vi "Main.vi"(11 "Module Admin":refnum<class "Delacor_lib_QMH_Cloneable Module Admin.lvclass">) -> ()   [LabVIEW 2020, in "Lock-in amplifier.lvlib"]
doc: "This template is based off of the Queued Message Handler design pattern and the Queued Message Handler project template that ships with LabVIEW.\n\nThe main difference is that the queue is private to this module and communication between modules is performed via Broadcast and Request events.\n\nRequest events are wrapped in public API methods and are handled in the Event Handling Loop (EHL) of this VI. Any module can register for Broadcast events sent by this module. The EHL generates messages based on user interface actions.\n\nThe Message Handling Loop (MHL) processes messages generated by the EHL, or by other messages. The messages are string values, so new messages can be added easily to the Message Cases case structure in the MHL. Each message cluster can also provide an optional value for Message Data, which is a variant that can be converted to whatever message-specific data is required.\n_____\nBased on DQMH Project Template 6.1.0.94.\n____\nPantherLAB Templates 1.0.0.1\nCopyright (c) 2022, PantherLAB\n____\nPantherLAB Templates 1.0.0.5\nCopyright (c) 2022, PantherLAB"
uses:
  Lock-in amplifier.lvlib
  <vilib>/Delacor/Delacor QMH/Libraries/Cloneable Module Admin_class/Delacor_lib_QMH_Cloneable Module Admin.lvclass
  C:/Program Files (x86)/National Instruments/LabVIEW 2020/vi.lib/Delacor/Delacor QMH/Libraries/Module Admin_class/Delacor_lib_QMH_Module Admin.lvclass
  Module Data--cluster.ctl
  Helper Loop Status--enum.ctl
  <vilib>/Delacor/Delacor QMH/Libraries/Cloneable Module Admin_class/Delacor_lib_QMH_Cloneable Module Admin.lvclass/Delacor_lib_QMH_Cloneable Module Admin.ctl
  <vilib>/Delacor/Delacor QMH/Libraries/Message Queue_class/Delacor_lib_QMH_Message Queue.lvclass/Delacor_lib_QMH_Message Queue.ctl
  Stop Argument--cluster.ctl
  <vilib>/Delacor/Delacor QMH/Libraries/Module Admin_class/Delacor_lib_QMH_Module Admin.lvclass/Delacor_lib_QMH_Module Admin.ctl
  Draw Panel into Subpanel Argument--cluster.ctl
  Remove Panel from Subpanel Argument--cluster.ctl
  <vilib>/Utility/miscctls.llb/LVPointTypeDef.ctl
  <vilib>/Delacor/Delacor QMH/Libraries/Cloneable Module Admin_class/Delacor_lib_QMH_Get Module ID.vi
  <vilib>/Delacor/Delacor QMH/Libraries/Message Queue_class/Delacor_lib_QMH_Enqueue Message (Single).vi
  <vilib>/Delacor/Delacor QMH/Libraries/Module Admin_class/Delacor_lib_QMH_Get External Launch.vi
  <vilib>/Utility/error.llb/Error Cluster From Error Code.vi
  <vilib>/ErrorRing/Error Ring.xnode
  <vilib>/Delacor/Delacor QMH/Libraries/Message Queue_class/Delacor_lib_QMH_Message Queue.lvclass
  Local Events/Local Events.lvlib
panel:
  out "error out":errorcluster
  out "Status":string
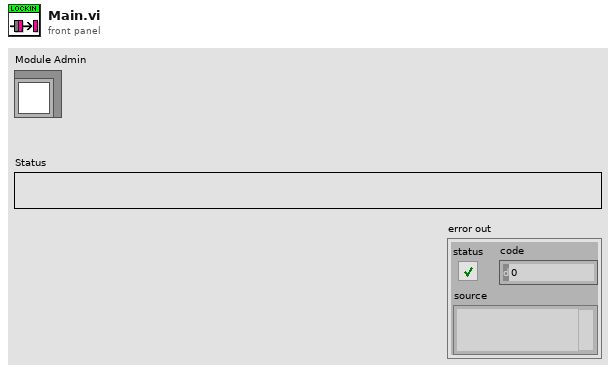
[diagram p1: front panel]
types:
  T1 = typedef "Lock-in amplifier.lvlib/Request Events--cluster.ctl" = cluster{"Stop Module":refnum<user-event>, "Show Panel":refnum<user-event>, "Hide Panel":refnum<user-event>, "Show Diagram":refnum<user-event>, "Get Module Execution Status":refnum<user-event>, "Draw Panel into Subpanel":refnum<user-event>, "Remove Panel from Subpanel":refnum<user-event>}
  T2 = typedef "Lock-in amplifier.lvlib/Local Events.lvlib/Local Events--cluster.ctl" = cluster{"Wake up Helper Loop":refnum<user-event>, "Put Helper Loop to Sleep":refnum<user-event>}
  T3 = typedef "Lock-in amplifier.lvlib/Module Data--cluster.ctl" = cluster{"Status":string, "SubPanel":refnum<vi>, "Panel Status":bool}
  T4 = typedef "Lock-in amplifier.lvlib/Helper Loop Status--enum.ctl" = enum16{"Awake", "Asleep"}
  T5 = enum32{"invalid lock state", "Not Locked", "Locked (No Password)", "Password-protected"}
  T6 = typedef "Lock-in amplifier.lvlib/Stop Argument--cluster.ctl" = cluster{"Module ID":i32, "Origin":string, "Exit via Stop Module Req?":bool, "Wait for Module to stop?":bool}
  T7 = typedef "Lock-in amplifier.lvlib/Draw Panel into Subpanel Argument--cluster.ctl" = cluster{"Module ID":i32, "Sub Panel":refnum<vi>}
  T8 = typedef "Lock-in amplifier.lvlib/Remove Panel from Subpanel Argument--cluster.ctl" = cluster{"Module ID":i32, "Boolean":bool}
  T9 = typedef "LVPointTypeDef.ctl" = cluster{"Horizontal":i16, "Vertical":i16}
  T10 = enum32{"Invalid", "Standard", "Closed", "Hidden", "Minimized", "Maximized"}
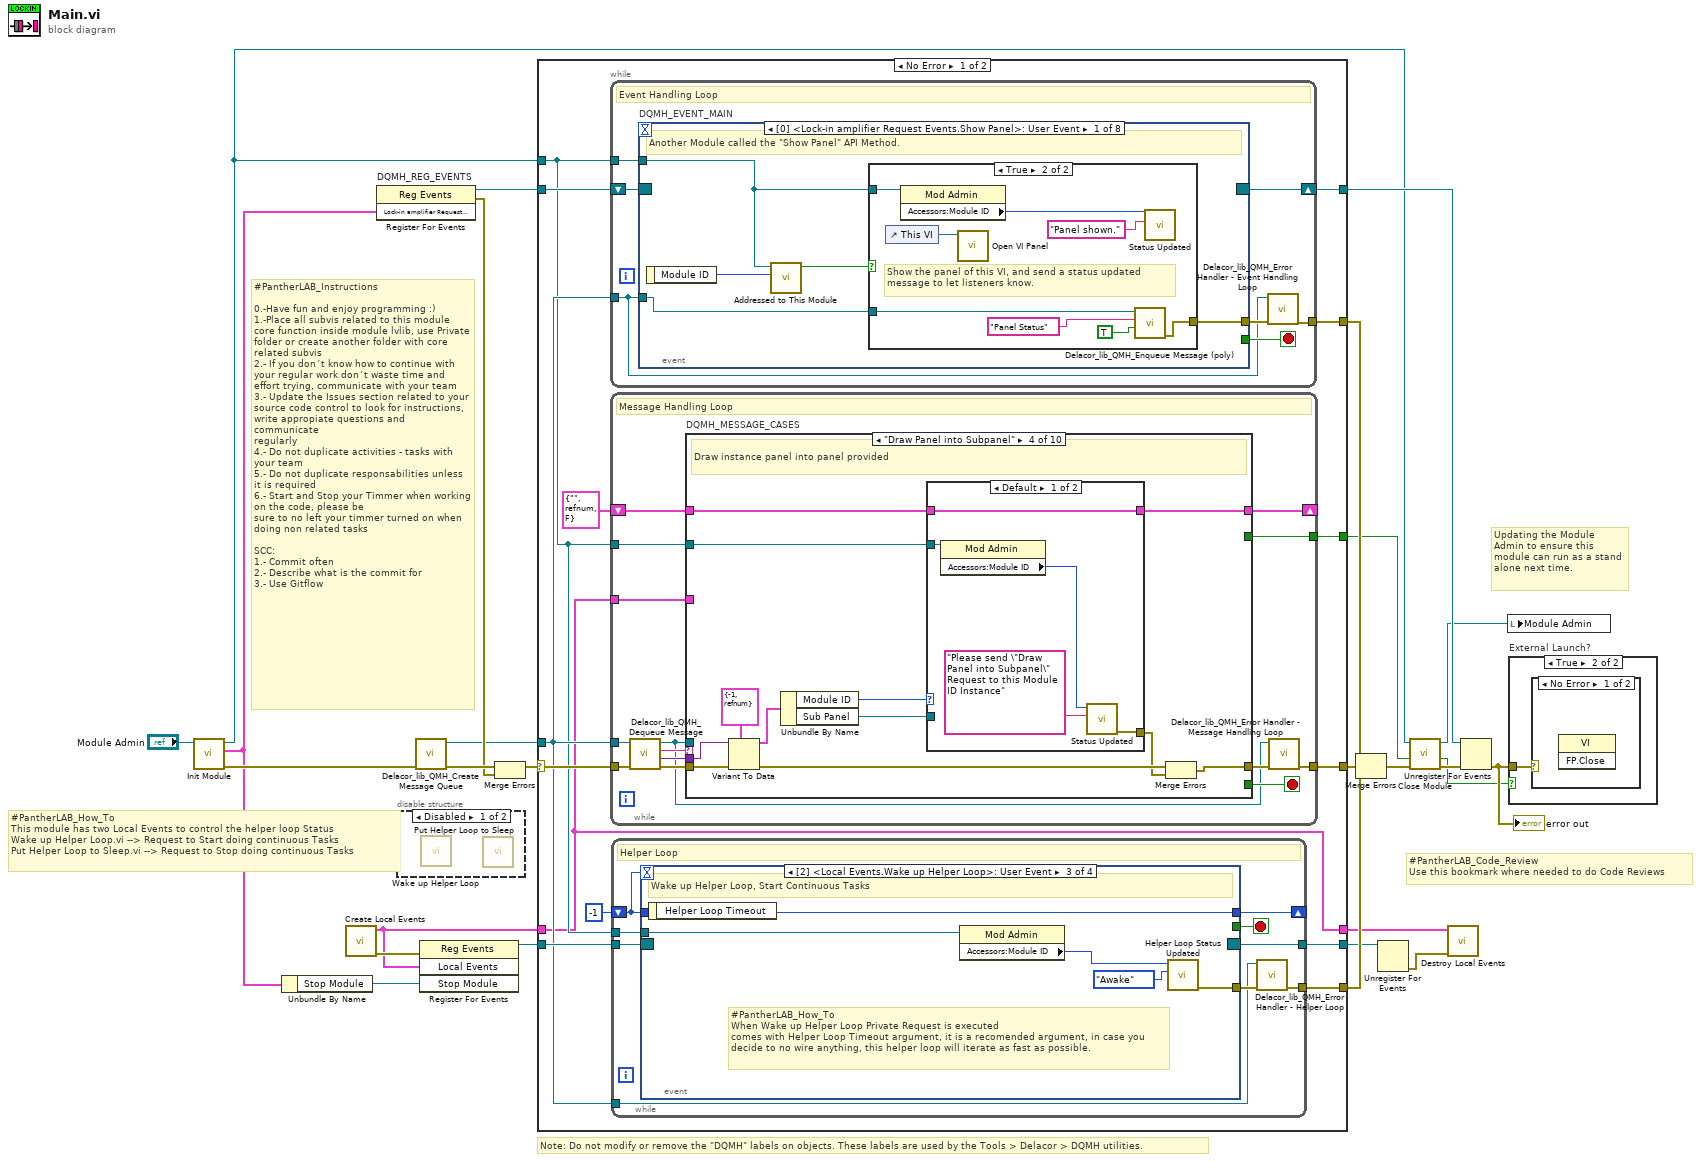
[diagram p0: block diagram]
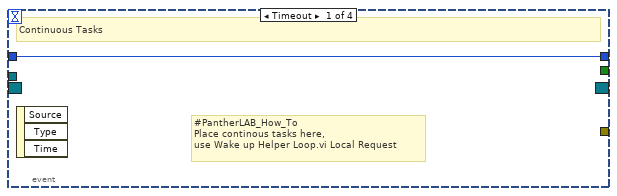
[diagram p3: hidden frame]
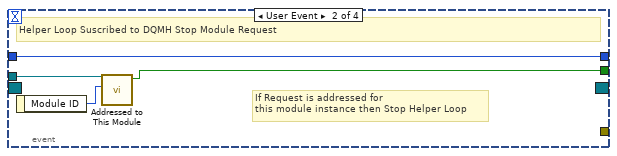
[diagram p4: hidden frame]
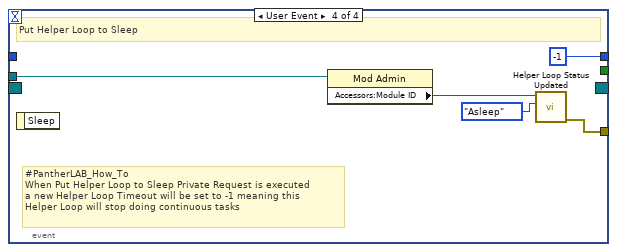
[diagram p5: hidden frame]
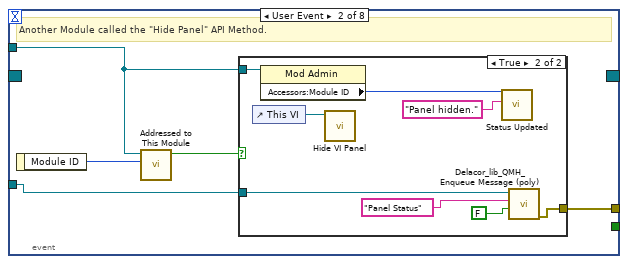
[diagram p7: hidden frame]
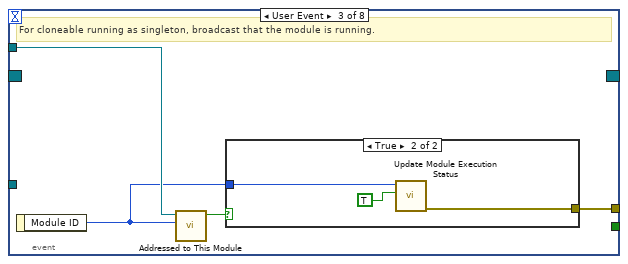
[diagram p9: hidden frame]
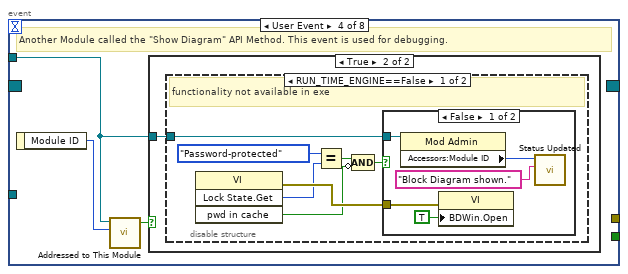
[diagram p11: hidden frame]
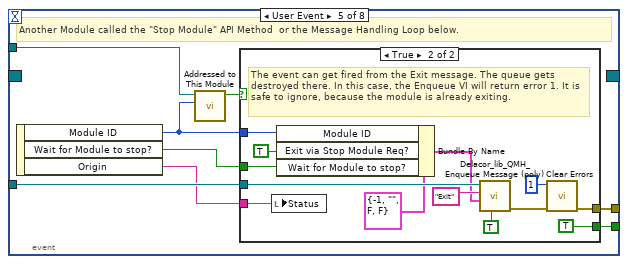
[diagram p15: hidden frame]
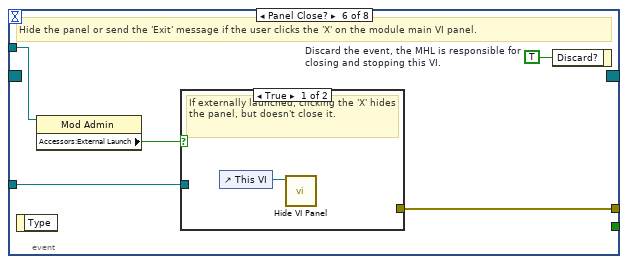
[diagram p17: hidden frame]
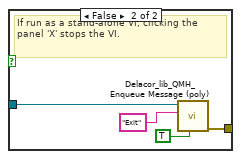
[diagram p18: hidden frame]
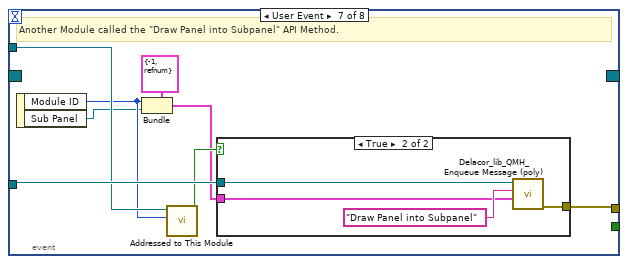
[diagram p19: hidden frame]
diagram:
  # "#PantherLAB_How_To\nThis module has two Local Events to control the helper loop Status\nWake up Helper Loop.vi --> Request to Start doing continuous Tasks\nPut Helper Loop to Sleep.vi --> Request to Stop doing continuous Tasks"
  # "#PantherLAB_Code_Review\nUse this bookmark where needed to do Code Reviews"
  # "#PantherLAB_Instructions\n\n0.-Have fun and enjoy programming :)\n1.-Place all subvis related to this module core function inside module lvlib, use Private folder or create another folder with core related subvis \n2.- If you don´t know how to continue with your regular work don´t waste time and effort trying, communicate with your team\n3.- Update the Issues section related to your source code control to look for instructions, write appropiate questions and communicate\nregularly\n4.- Do not duplicate activities - tasks with your team\n5.- Do not duplicate responsabilities unless it is required\n6.- Start and Stop your Timmer when working on the code, please be\nsure to no left your timmer turned on when doing non related tasks\n\nSCC:\n1.- Commit often\n2.- Describe what is the commit for\n3.- Use Gitflow"
  # "Note: Do not modify or remove the \"DQMH\" labels on objects. These labels are used by the Tools > Delacor > DQMH utilities."
  # "Updating the Module Admin to ensure this module can run as a stand alone next time."
  n1 = call "Init Module.vi"("Cloneable Module Admin in"="Module Admin") -> ("error out"=w23:errorcluster, "Lock-in amplifier Request Events"=w4:T1, "Cloneable Module Admin out"=w10:refnum<class "Delacor_lib_QMH_Cloneable Module Admin.lvclass">)  [unwired: 8 in]
  n2 = Unbundle By Name(w4) -> ("Stop Module"=w3:refnum<user-event>)
  n3 = call "Create Local Events.vi"() -> ("error out"=w16:errorcluster, "Local Events"=w2:T2)  [unwired: 10 in]
  n4 = register-events "DQMH_REG_EVENTS"(w4) -> (reference out=w13:refnum<event-registration>, error out=w18:errorcluster)  [unwired: 2 in]
  n5 = disable-structure shown="Disabled" {
    frame Disabled {
      n6 = call "Wake up Helper Loop.vi"() -> ()  [unwired: 11 in, 1 out]
      n7 = call "Put Helper Loop to Sleep.vi"() -> ()  [unwired: 11 in, 1 out]
    }
    frame Enabled {
    }
  }
  n8 = call <vilib>:"Delacor_lib_QMH_Create Message Queue.vi"("error in"=w23) -> ("error out"=w20:errorcluster, "Message Queue"=w12:refnum<class "Delacor_lib_QMH_Message Queue.lvclass">)  [unwired: 9 in]
  n9 = register-events(error in=w16, w2, w3) -> (reference out=w5:refnum<event-registration>)  [unwired: 1 in, 1 out]
  n10 = Merge Errors(w20, w18) -> (w19:errorcluster)
  n11 = case shown="No Error" w19 {
    selector: w19 -> [w38 w326]
    tunnel: [w40 w325] -> w24
    tunnel: [w36 w324] -> w14
    tunnel: w13 -> [w34 w324]
    tunnel: w12 -> [w29 w317]
    tunnel: [w39 _] -> w25
    tunnel: w10 -> [w28 w320]
    tunnel: [w33 _] -> w8
    tunnel: [w32 w316] -> w6
    tunnel: w5 -> [w31 w316]
    tunnel: [w37 _] -> w17
    tunnel: w2 -> [w27 w315]
    tunnel: [w27 w315] -> w1
    frame No Error {
      n12 = while {
        tunnel: w29 -> [w65]
        shift-right: [w68] -> w36
        shift-left: w34 -> [w69]
        tunnel: [w70] -> w39
        tunnel: w28 -> [w66]
        stop <- w67 stop-if-true
        # "Event Handling Loop"
        n13 = event "DQMH_EVENT_MAIN" shown="[0] <Lock-in amplifier Request Events.Show Panel>: User Event" {
          selector: w69 -> [_ _ _ _ _ _ _ _]
          dyn-events: [_ _ _ _ _ _ _ _] -> w68
          timeout: _ -> [_ _ _ _ _ _ _ _]
          tunnel: [_ _ _ _ w124 _ _ _] -> w67
          tunnel: w65 -> [w72 w85 _ _ w127 w143 w158 w170]
          tunnel: [w76 w89 w101 _ w128 w146 w159 w171] -> w71
          tunnel: w66 -> [w73 w86 w99 w105 w126 w144 w156 w168]
          event User Event {
            # "Another Module called the \"Show Panel\" API Method."
            n14 = event-data() -> ("Module ID"=w74:i32)  [unwired: 1 in]
            n15 = call "Addressed to This Module.vi"("Module ID from Argument"=w74, "Module Admin"=w73) -> ("Addressed to this instance?"=w75:bool)  [unwired: 8 in, 1 out]
            n16 = case shown="True" w75 {
              tunnel: w73 -> [_ w81]
              tunnel: w72 -> [_ w79]
              tunnel: [_ w84] -> w76
              frame False {
              }
              frame True {
                # "Show the panel of this VI, and send a status updated message to let listeners know."
                n17 = control-ref of="This VI"() -> (w83:refnum<vi>)
                n18 = property class="Mod Admin"(reference=w81) -> ("Accessors:Module ID"=w80:i32)  [unwired: 1 in, 2 out]
                n19 = call "Open VI Panel.vi"("VI"=w83) -> ()  [unwired: 10 in, 1 out]
                n20 = call-poly <vilib>:"Delacor_lib_QMH_Enqueue Message (poly).vi"("Message Data"=TRUE, "Message"="Panel Status" ("format string"), "Message Queue in"=w79) -> ("error out"=w84:errorcluster)  [unwired: 7 in, 1 out]
                n21 = call "Status Updated.vi"("Status"="Panel shown." ("format string"), "Module ID"=w80) -> ()  [unwired: 9 in, 1 out]
              }
            }
          }
          event User Event {
            # "Another Module called the \"Hide Panel\" API Method."
            n22 = event-data() -> ("Module ID"=w87:i32)  [unwired: 1 in]
            n23 = call "Addressed to This Module.vi"("Module ID from Argument"=w87, "Module Admin"=w86) -> ("Addressed to this instance?"=w88:bool)  [unwired: 8 in, 1 out]
            n24 = case shown="True" w88 {
              tunnel: w86 -> [_ w94]
              tunnel: w85 -> [_ w90]
              tunnel: [_ w97] -> w89
              frame False {
              }
              frame True {
                n25 = control-ref of="This VI"() -> (w96:refnum<vi>)
                n26 = property class="Mod Admin"(reference=w94) -> ("Accessors:Module ID"=w93:i32)  [unwired: 1 in, 2 out]
                n27 = call "Hide VI Panel.vi"("VI"=w96) -> ()  [unwired: 10 in, 1 out]
                n28 = call "Status Updated.vi"("Status"="Panel hidden." ("format string"), "Module ID"=w93) -> ()  [unwired: 9 in, 1 out]
                n29 = call-poly <vilib>:"Delacor_lib_QMH_Enqueue Message (poly).vi"("Message Data"=FALSE, "Message"="Panel Status" ("format string"), "Message Queue in"=w90) -> ("error out"=w97:errorcluster)  [unwired: 7 in, 1 out]
              }
            }
          }
          event User Event {
            # "For cloneable running as singleton, broadcast that the module is running."
            n30 = event-data() -> ("Module ID"=w98:i32)  [unwired: 1 in]
            n31 = call "Addressed to This Module.vi"("Module ID from Argument"=w98, "Module Admin"=w99) -> ("Addressed to this instance?"=w100:bool)  [unwired: 8 in, 1 out]
            n32 = case shown="True" w100 {
              tunnel: [_ w104] -> w101
              tunnel: w98 -> [_ w103]
              frame False {
              }
              frame True {
                n33 = call "Update Module Execution Status.vi"("Running?"=TRUE, "Module ID"=w103) -> ("error out"=w104:errorcluster)  [unwired: 9 in]
              }
            }
          }
          event User Event {
            # "Another Module called the \"Show Diagram\" API Method. This event is used for debugging."
            n34 = event-data() -> ("Module ID"=w106:i32)  [unwired: 1 in]
            n35 = call "Addressed to This Module.vi"("Module ID from Argument"=w106, "Module Admin"=w105) -> ("Addressed to this instance?"=w107:bool)  [unwired: 8 in, 1 out]
            n36 = case shown="True" w107 {
              tunnel: w105 -> [_ w108]
              frame False {
              }
              frame True {
                n37 = disable-structure shown="RUN_TIME_ENGINE==False" {
                  disable-tunnel: w108 -> [w109 _]
                  frame condition #0 (active) {
                    # "functionality not available in exe"
                    n38 = invoke class="VI" method="Lock State.Get"() -> (error out=w115:errorcluster, "Get Lock State"=w114:T5, "pwd in cache"=w111:bool)  [unwired: 4 in, 1 out]
                    n39 = Equal?(x=T5."Password-protected", y=w114) -> (x = y?=w112:bool)
                    n40 = Compound Arithmetic op=AND(w112, invert w111) -> (w110:bool)
                    n41 = case shown="False" w110 {
                      tunnel: w115 -> [w120 _]
                      tunnel: w109 -> [w117 _]
                      frame False {
                        n42 = property class="Mod Admin"(reference=w117) -> ("Accessors:Module ID"=w116:i32)  [unwired: 1 in, 2 out]
                        n43 = property class="VI"(error in=w120, "BDWin.Open"=TRUE ("Block Diagram Window:Open")) -> ()  [unwired: 1 in, 2 out]
                        n44 = call "Status Updated.vi"("Status"="Block Diagram shown." ("format string"), "Module ID"=w116) -> ()  [unwired: 9 in, 1 out]
                      }
                      frame True {
                        # "Password-protected VI, and the password is not in the cache. Do not show the diagram."
                      }
                    }
                  }
                  frame condition #1 {
                  }
                }
              }
            }
          }
          event User Event {
            # "Another Module called the \"Stop Module\" API Method  or the Message Handling Loop below."
            n45 = event-data() -> ("Module ID"=w122:i32, "Wait for Module to stop?"=w123:bool, "Origin"=w121:string)  [unwired: 1 in]
            n46 = call "Addressed to This Module.vi"("Module ID from Argument"=w122, "Module Admin"=w126) -> ("Addressed to this instance?"=w125:bool)  [unwired: 8 in, 1 out]
            n47 = case shown="True" w125 {
              tunnel: [_ w140] -> w128
              tunnel: w127 -> [_ w136]
              tunnel: [_ TRUE] -> w124
              tunnel: w123 -> [_ w131]
              tunnel: w122 -> [_ w133]
              tunnel: w121 -> [_ w129]
              frame False {
              }
              frame True {
                # "The event can get fired from the Exit message. The queue gets destroyed there. In this case, the Enqueue VI will return error 1. It is safe to ignore, because the module is already exiting."
                n48 = local write "Status"(w129) -> ()
                n49 = Bundle By Name(cluster=T6 {"Module ID"=-1, "Origin"="", "Exit via Stop Module Req?"=FALSE, "Wait for Module to stop?"=FALSE} ("Stop Argument"), "Module ID"=w133, "Exit via Stop Module Req?"=TRUE, "Wait for Module to stop?"=w131) -> (w130:T6)
                n50 = call-poly <vilib>:"Delacor_lib_QMH_Enqueue Message (poly).vi"("Priority Message? (F)"=TRUE, "Message Data"=w130, "Message"="Exit", "Message Queue in"=w136) -> ("error out"=w141:errorcluster)  [unwired: 6 in, 1 out]
                n51 = call <vilib>:"Clear Errors.vi"("error in (no error)"=w141, "specific error code to clear (0: all)"=1) -> ("error out"=w140:errorcluster)  [unwired: 4 in, 1 out]
              }
            }
          }
          event Panel Close? {
            w145 = TRUE  # Discard the event, the MHL is responsible for closing and stopping this VI.
            # "Hide the panel or send the 'Exit' message if the user clicks the 'X' on the module main VI panel."
            n52 = event-data() -> ()  [unwired: 1 in, 1 out]
            n53 = property class="Mod Admin"(reference=w144) -> ("Accessors:External Launch"=w142:bool)  [unwired: 1 in, 2 out]
            n54 = case shown="True" w142 {
              tunnel: w143 -> [_ w150]
              tunnel: [_ w151] -> w146
              frame True {
                # "If externally launched, clicking the 'X' hides the panel, but doesn't close it."
                n55 = control-ref of="This VI"() -> (w147:refnum<vi>)
                n56 = call "Hide VI Panel.vi"("VI"=w147) -> ()  [unwired: 10 in, 1 out]
              }
              frame False {
                # "If run as a stand-alone VI, clicking the panel 'X' stops the VI."
                n57 = call-poly <vilib>:"Delacor_lib_QMH_Enqueue Message (poly).vi"("Priority Message? (F)"=TRUE, "Message"="Exit", "Message Queue in"=w150) -> ("error out"=w151:errorcluster)  [unwired: 7 in, 1 out]
              }
            }
            n58 = event-data("Discard?"=w145) -> ()  [unwired: 1 in, 1 out]
          }
          event User Event {
            # "Another Module called the \"Draw Panel into Subpanel\" API Method."
            n59 = event-data() -> ("Module ID"=w153:i32, "Sub Panel"=w152:refnum<vi>)  [unwired: 1 in]
            n60 = Bundle(cluster=T7 {"Module ID"=-1, "Sub Panel"=refnum} ("Draw Panel into Subpanel Argument"), "Module ID"=w153, "Sub Panel"=w152) -> (w154:T7)
            n61 = call "Addressed to This Module.vi"("Module ID from Argument"=w153, "Module Admin"=w156) -> ("Addressed to this instance?"=w157:bool)  [unwired: 8 in, 1 out]
            n62 = case shown="True" w157 {
              tunnel: w158 -> [_ w162]
              tunnel: w154 -> [_ w160]
              tunnel: [_ w163] -> w159
              frame False {
              }
              frame True {
                n63 = call-poly <vilib>:"Delacor_lib_QMH_Enqueue Message (poly).vi"("Message Data"=w160, "Message"="Draw Panel into Subpanel", "Message Queue in"=w162) -> ("error out"=w163:errorcluster)  [unwired: 7 in, 1 out]
              }
            }
          }
          event User Event {
            # "Another Module called the \"Remove Panel from Subpanel\" API Method."
            n64 = event-data() -> ("Module ID"=w165:i32, "Boolean"=w164:bool)  [unwired: 1 in]
            n65 = Bundle(cluster=T8 {"Module ID"=-1, "Boolean"=FALSE} ("Remove Panel from Subpanel Argument"), "Module ID"=w165, "Boolean"=w164) -> (w166:T8)
            n66 = call "Addressed to This Module.vi"("Module ID from Argument"=w165, "Module Admin"=w168) -> ("Addressed to this instance?"=w169:bool)  [unwired: 8 in, 1 out]
            n67 = case shown="True" w169 {
              tunnel: w170 -> [_ w174]
              tunnel: w166 -> [_ w172]
              tunnel: [_ w175] -> w171
              frame False {
              }
              frame True {
                n68 = call-poly <vilib>:"Delacor_lib_QMH_Enqueue Message (poly).vi"("Message Data"=w172, "Message"="Remove Panel from Subpanel", "Message Queue in"=w174) -> ("error out"=w175:errorcluster)  [unwired: 7 in, 1 out]
              }
            }
          }
        }
        n69 = call-dynamic "Delacor_lib_QMH_Error Handler - Event Handling Loop.vi"("error in"=w71, "Message Queue in"=w65) -> ("dup error in"=w70:errorcluster)  [unwired: 8 in, 1 out]
      }
      n70 = while {
        tunnel: w29 -> [w180]
        shift-right: [w184] -> _
        shift-left: T3 {"Status"="", "SubPanel"=refnum, "Panel Status"=FALSE} ("Data Cluster") -> [w185]
        tunnel: w38 -> [w188]
        tunnel: [w186] -> w40
        tunnel: w28 -> [w178]
        tunnel: [w177] -> w33
        tunnel: w27 -> [w176]
        stop <- w183 stop-if-true
        # "Message Handling Loop"
        n71 = call-dynamic "Delacor_lib_QMH_Dequeue Message.vi"("error in"=w188, "Message Queue in"=w180) -> ("error out"=w187:errorcluster, "Message Data"=w181:variant, "Message"=w182:string, "Message Queue out"=w179:refnum<class "Delacor_lib_QMH_Message Queue.lvclass">)  [unwired: 6 in]
        n72 = case "DQMH_MESSAGE_CASES" shown="\"Draw Panel into Subpanel\"" w182 {
          selector: w182 -> [_ _ _ _ _ _ _ _ _ w302]
          tunnel: w179 -> [_ _ _ _ _ _ _ w266 w292 _]
          tunnel: w187 -> [w208 w212 w219 w231 w250 w262 w264 w275 w298 w304]
          tunnel: [w206 w212 w218 w229 w249 w261 w264 w271 w295 w305] -> w189
          tunnel: w185 -> [w199 w211 w217 w222 w244 w260 w263 w270 w283 w303]
          tunnel: [w198 w211 w214 w221 w244 w260 w263 w270 w283 w303] -> w184
          tunnel: [_ _ _ _ _ _ _ _ w291 _] -> w183
          tunnel: w181 -> [_ _ w216 w227 w248 _ _ w269 w289 _]
          tunnel: w178 -> [w193 _ _ w220 w243 _ _ w268 w285 w300]
          tunnel: [_ _ _ _ _ _ _ _ w287 _] -> w177
          tunnel: w176 -> [_ _ _ _ _ _ _ _ _ _]
          frame "Initialize" {
            w190 = "Initial Message" ("Initial Message")
            # "#CodeNeeded - Initialize the appearance of the front panel."
            # "#CodeNeeded - Initialize your state data here."
            # "Initialize - Any operation that needs to be done before the module can receive messages. Synchronize Caller Events.vi will inform Start Module.vi that the module has launched and is ready to receive messages. Module Did Init.vi will broadcast that the module initialized."
            n73 = call "Synchronize Caller Events.vi"("error in (no error)"=w208, "Module Admin"=w193) -> ("error out"=w207:errorcluster, "Module Admin out"=w192:refnum<class "Delacor_lib_QMH_Cloneable Module Admin.lvclass">)  [unwired: 8 in]
            n74 = property class="Mod Admin"(reference=w192) -> ("Accessors:Module ID"=w195:i32, "Accessors:External Launch"=w194:bool)  [unwired: 1 in, 2 out]
            n75 = call "Module Name--constant.vi"("Module ID"=w195) -> ("Module Name"=w203:string)  [unwired: 10 in]
            n76 = property class="VI"("Front Panel.Title"=w203) -> (reference out=w205:refnum<vi>, error out=w210:errorcluster)  [unwired: 2 in]
            n77 = Select(t=T10."Hidden" ("State"), s=w194, f=T10."Standard" ("State")) -> (s? t:f=w200:T10)
            n78 = invoke class="VI" method="FP.Open"(reference=w205, error in=w210, "State"=w200) -> (reference out=w204:refnum<vi>, error out=w209:errorcluster)  [unwired: 2 in, 3 out]
            n79 = call "Module Name--constant.vi"("Module ID"=w195) -> ("Module Name"=w196:string)  [unwired: 10 in]
            n80 = Bundle By Name(cluster=w199, "Status"=w190) -> (w198:T3)
            n81 = invoke class="VI" method="FP.Center"(reference=w204, error in=w209) -> ()  [unwired: 1 in, 3 out]
            n82 = property on="Pane" class="Pane"("Origin"=T9 {"Horizontal"=0, "Vertical"=0}) -> ()  [unwired: 2 in, 2 out]
            n83 = call "Module Did Init.vi"("error in (no error)"=w207, "Initialized?"=TRUE, "Origin"=w196, "Module ID"=w195) -> ("error out"=w206:errorcluster)  [unwired: 7 in]
            "Status" <- w190
          }
          frame "---Module Specific---" {
            # "Separator -- The following cases handle messages specific to this Module."
          }
          frame "Panel Status" {
            n84 = Variant To Data(error in=w219, type=TRUE, Variant=w216) -> (data=w213:bool, error out=w218:errorcluster)
            n85 = Bundle By Name(cluster=w217, "Panel Status"=w213) -> (w214:T3)
          }
          frame "Draw Panel into Subpanel" {
            # "Draw instance panel into panel provided"
            n86 = Variant To Data(error in=w231, type=T7 {"Module ID"=-1, "Sub Panel"=refnum} ("Draw Panel into Subpanel Argument"), Variant=w227) -> (data=w225:T7, error out=w230:errorcluster)
            n87 = Unbundle By Name(w225) -> ("Module ID"=w223:i32, "Sub Panel"=w224:refnum<vi>)
            n88 = case shown="Default" w223 {
              tunnel: w224 -> [_ w241]
              tunnel: [w236 w242] -> w228
              tunnel: w222 -> [w234 w239]
              tunnel: [w234 w238] -> w221
              tunnel: w220 -> [w233 _]
              frame Default {
                n89 = property class="Mod Admin"(reference=w233) -> ("Accessors:Module ID"=w232:i32)  [unwired: 1 in, 2 out]
                n90 = call "Status Updated.vi"("Status"="Please send \"Draw Panel into Subpanel\" Request to this Module ID Instance", "Module ID"=w232) -> ("error out"=w236:errorcluster)  [unwired: 9 in]
              }
              frame 0.. {
                n91 = control-ref of="This VI"() -> (w240:refnum<vi>)
                n92 = call "Draw Panel into Subpanel Procedure.vi"("SubPanel in"=w241, "This VI"=w240) -> ("error out"=w242:errorcluster, "SubPanel out"=w237:refnum<vi>)  [unwired: 8 in]
                n93 = Bundle By Name(cluster=w239, "SubPanel"=w237) -> (w238:T3)
              }
            }
            n94 = Merge Errors(w230, w228) -> (w229:errorcluster)
          }
          frame "Remove Panel from Subpanel" {
            # "Remove panel from subpanel"
            n95 = Variant To Data(error in=w250, type=T8 {"Module ID"=-1, "Boolean"=FALSE} ("Remove Panel from Subpanel Argument"), Variant=w248) -> (data=w246:T8, error out=w249:errorcluster)
            n96 = Unbundle By Name(w246) -> ("Module ID"=w245:i32)
            n97 = case shown="-1" w245 {
              tunnel: w244 -> [w254 _]
              tunnel: w243 -> [_ w258]
              frame Default {
                n98 = Unbundle By Name(w254) -> ("Panel Status"=w252:bool, "SubPanel"=w253:refnum<vi>)
                n99 = control-ref of="This VI"() -> (w251:refnum<vi>)
                n100 = case shown="True" w252 {
                  tunnel: w251 -> [w255 w256]
                  frame False {
                    n101 = call "Hide VI Panel.vi"("VI"=w255) -> ()  [unwired: 10 in, 1 out]
                  }
                  frame True {
                    n102 = call "Open VI Panel.vi"("VI"=w256) -> ()  [unwired: 10 in, 1 out]
                  }
                }
                n103 = invoke class="SubPnl" method="Remove VI"(reference=w253) -> ()  [unwired: 2 in, 3 out]
              }
              frame -1 {
                n104 = property class="Mod Admin"(reference=w258) -> ("Accessors:Module ID"=w257:i32)  [unwired: 1 in, 2 out]
                n105 = call "Status Updated.vi"("Status"="Please send \"Remove panel from subpanel\" Request to this Module ID Instance", "Module ID"=w257) -> ()  [unwired: 9 in, 1 out]
              }
            }
          }
          frame "---Copy This Frame---" {
            # "Duplicate this frame when creating new messages.  Change this comment in the duplicated frame to describe this message."
            n106 = Merge Errors(w262) -> (w261:errorcluster)
          }
          frame "---Exit and Error Handling---" {
            # "Separator - the following cases handle errors and exit messages."
          }
          frame "Error" {
            # "#CodeRecommended - If you ever change the name of this \"Error\" message, you'll need to update the name in the Check Loop Error.vi as well."
            # "#CodeRecommended - If the module is running in standalone mode (External Launch = FALSE), this code will pop up an error dialog and call the 'Exit' message if an error occurs. Add more fine-grained error handling here."
            # "Error - Check the error message data and respond accordingly. This message is sent by the \"Error Handler\" VIs at the end of each loop in this application."
            n107 = property class="Mod Admin"(reference=w268) -> ("Accessors:External Launch"=w267:bool, "Accessors:Module ID"=w265:i32)  [unwired: 1 in, 2 out]
            n108 = Variant To Data(error in=w275, type=errorcluster {"status"=FALSE, "code"=0, "source"=""} ("error constant"), Variant=w269) -> (data=w276:errorcluster, error out=w273:errorcluster)
            n109 = call "Error Reported.vi"("Error"=w276, "Module ID"=w265) -> ()  [unwired: 9 in, 1 out]
            n110 = case shown="False" w267 {
              tunnel: [w281 _] -> w272
              tunnel: w266 -> [w279 _]
              tunnel: w276 -> [w280 _]
              frame False {
                # "If the module is running standalone, then pop up an error dialog and call the \"Exit\" message."
                n111 = call <vilib>:"Simple Error Handler.vi"("error in (no error)"=w280) -> ()  [unwired: 4 in, 5 out]
                n112 = call-poly <vilib>:"Delacor_lib_QMH_Enqueue Message (poly).vi"("Priority Message? (F)"=TRUE, "Message"="Exit", "Message Queue in"=w279) -> ("error out"=w281:errorcluster)  [unwired: 7 in, 1 out]
              }
              frame True {
                # "If the module was launched externally, calling the Error Reported broadcast VI is the only action performed by the \"Error\" message. The module's caller can then process the error appropriately."
              }
            }
            n113 = Merge Errors(w273, w272) -> (w271:errorcluster)
            n114 = local write "error out"(w271) -> ()
          }
          frame "Exit" {
            w290 = 91  # 91: not all Exit messages will have an argument
            w291 = TRUE  # Stop the VI
            # "Release the message queue reference"
            # "Exit - Exit the application."
            n115 = Variant To Data(error in=w298, type=T6 {"Module ID"=-1, "Origin"="", "Exit via Stop Module Req?"=FALSE, "Wait for Module to stop?"=FALSE} ("Stop Argument"), Variant=w289) -> (data=w286:T6, error out=w293:errorcluster)
            n116 = call <vilib>:"Clear Errors.vi"("error in (no error)"=w293, "specific error code to clear (0: all)"=w290) -> ("error out"=w297:errorcluster)  [unwired: 4 in, 1 out]
            n117 = Unbundle By Name(w283) -> ("SubPanel"=w282:refnum<vi>)
            n118 = invoke class="SubPnl" method="Remove VI"(reference=w282) -> ()  [unwired: 2 in, 3 out]
            n119 = control-ref of="This VI"() -> (w284:refnum<vi>)
            n120 = call-dynamic "Delacor_lib_QMH_Release Message Queue.vi"("error in"=w297, "Message Queue"=w292) -> ("error out"=w296:errorcluster)  [unwired: 9 in]
            n121 = call "Handle Exit.vi"("Stop Argument"=w286, "Module Admin in"=w285, "VI reference"=w284) -> ("error out"=w294:errorcluster, "Wait for Stop?"=w287:bool)  [unwired: 7 in]
            n122 = Merge Errors(w296, w294) -> (w295:errorcluster)
          }
          frame Default {
            # "'Default' case only runs if there is a message that isn't defined in any of the other cases.  Output a programming error."
            n123 = property class="Mod Admin"(reference=w300) -> ("Accessors:Module ID"=w299:i32)  [unwired: 1 in, 2 out]
            n124 = call "Module Name--constant.vi"("Module ID"=w299) -> ("Module Name"=w301:string)  [unwired: 10 in]
            n125 = xnode "Error Ring"("parameter 0"=w302, "parameter 1"=w301) -> ("error out"=w306:errorcluster)
            n126 = Merge Errors(w304, w306) -> (w305:errorcluster)
          }
        }
        n127 = call-dynamic "Delacor_lib_QMH_Error Handler - Message Handling Loop.vi"("error in"=w189, "Message Queue in"=w179) -> ("dup error in"=w186:errorcluster)  [unwired: 8 in, 1 out]
      }
      n128 = while {
        tunnel: w29 -> [w43]
        tunnel: w31 -> [w47]
        shift-right: [w45] -> _
        shift-left: -1 ("Helper Loop Timeout") -> [w46]
        tunnel: [w44] -> w32
        tunnel: [w49] -> w37
        tunnel: w28 -> [w41]
        stop <- w42 stop-if-true
        # "Helper Loop"
        n129 = event shown="[2] <Local Events.Wake up Helper Loop>: User Event" {
          selector: w47 -> [_ _ _ _]
          dyn-events: [_ _ _ _] -> w44
          timeout: w46 -> [_ _ _ _]
          tunnel: w46 -> [w50 w54 _ _]
          tunnel: [w50 w54 w55 -1 ("Helper Loop Timeout")] -> w45
          tunnel: [_ w51 _ _] -> w42
          tunnel: w41 -> [_ w53 w58 w63]
          tunnel: [_ _ w59 w64] -> w48
          event Timeout {
            # "#PantherLAB_How_To\nPlace continous tasks here,\nuse Wake up Helper Loop.vi Local Request"
            # "Continuous Tasks"
            n130 = event-data() -> ()  [unwired: 1 in, 3 out]
          }
          event User Event {
            # "If Request is addressed for\nthis module instance then Stop Helper Loop"
            # "Helper Loop Suscribed to DQMH Stop Module Request"
            n131 = event-data() -> ("Module ID"=w52:i32)  [unwired: 1 in]
            n132 = call "Addressed to This Module.vi"("Module ID from Argument"=w52, "Module Admin"=w53) -> ("Addressed to this instance?"=w51:bool)  [unwired: 8 in, 1 out]
          }
          event User Event {
            # "#PantherLAB_How_To\nWhen Wake up Helper Loop Private Request is executed\ncomes with Helper Loop Timeout argument, it is a recomended argument, in case you decide to no wire anything, this helper loop will iterate as fast as possible."
            # "Wake up Helper Loop, Start Continuous Tasks"
            n133 = event-data() -> ("Helper Loop Timeout"=w55:i32)  [unwired: 1 in]
            n134 = property class="Mod Admin"(reference=w58) -> ("Accessors:Module ID"=w56:i32)  [unwired: 1 in, 2 out]
            n135 = call "Helper Loop Status Updated.vi"("Helper Loop Status"=Helper_Loop_Status--enum."Awake", "Module ID"=w56) -> ("error out"=w59:errorcluster)  [unwired: 9 in]
          }
          event User Event {
            # "#PantherLAB_How_To\nWhen Put Helper Loop to Sleep Private Request is executed\na new Helper Loop Timeout will be set to -1 meaning this\nHelper Loop will stop doing continuous tasks"
            # "Put Helper Loop to Sleep"
            n136 = event-data() -> ()  [unwired: 1 in, 1 out]
            n137 = property class="Mod Admin"(reference=w63) -> ("Accessors:Module ID"=w60:i32)  [unwired: 1 in, 2 out]
            n138 = call "Helper Loop Status Updated.vi"("Helper Loop Status"=Helper_Loop_Status--enum."Asleep", "Module ID"=w60) -> ("error out"=w64:errorcluster)  [unwired: 9 in]
          }
        }
        n139 = call-dynamic "Delacor_lib_QMH_Error Handler - Helper Loop.vi"("error in"=w48, "Message Queue in"=w43) -> ("dup error in"=w49:errorcluster)  [unwired: 8 in, 1 out]
      }
    }
    frame Error {
      n140 = call "Synchronize Caller Events.vi"("Module Admin"=w320) -> ("Module Admin out"=w319:refnum<class "Delacor_lib_QMH_Cloneable Module Admin.lvclass">)  [unwired: 9 in, 1 out]
      n141 = property class="Mod Admin"(reference=w319) -> ("Accessors:Module ID"=w318:i32)  [unwired: 1 in, 2 out]
      n142 = call-dynamic "Delacor_lib_QMH_Release Message Queue.vi"("error in"=w326, "Message Queue"=w317) -> ("error out"=w325:errorcluster)  [unwired: 9 in]
      n143 = call "Module Name--constant.vi"("Module ID"=w318) -> ("Module Name"=w323:string)  [unwired: 10 in]
      n144 = Format Into String(format string="An error occurred during initialization. %s is no longer running.", w323) -> (resulting string=w321:string)  [unwired: 2 in, 1 out]
      n145 = call "Error Reported.vi"("Additional Information"=w321, "Error"=w325, "Module ID"=w318) -> ()  [unwired: 8 in, 1 out]
    }
  }
  n146 = Merge Errors(w25, w24, w17) -> (w26:errorcluster)
  n147 = Unregister For Events(event registration refnum=w6) -> (error out=w15:errorcluster)  [unwired: 1 in]
  n148 = call "Close Module.vi"("error in"=w26, "Wait for stop?"=w8, "Module Admin in"=w10) -> ("error out"=w22:errorcluster, "External Launch"=w7:bool, "Module Admin out"=w9:refnum<class "Delacor_lib_QMH_Cloneable Module Admin.lvclass">)  [unwired: 6 in]
  n149 = call "Destroy Local Events.vi"("error in"=w15, "Local Events"=w1) -> ()  [unwired: 9 in, 1 out]
  n150 = Unregister For Events(event registration refnum=w14, error in=w22) -> (error out=w21:errorcluster)
  "error out" <- w21
  n151 = local write "Module Admin"(w9) -> ()
  n152 = case "External Launch?" shown="True" w7 {
    tunnel: w21 -> [_ w327]
    frame False {
    }
    frame True {
      n153 = case shown="No Error" w327 {
        frame No Error {
          n154 = invoke class="VI" method="FP.Close"() -> ()  [unwired: 3 in, 3 out]
        }
        frame Error {
          n155 = invoke class="VI" method="FP.Open"("Activate"=TRUE ("Activate?")) -> ()  [unwired: 4 in, 5 out]
        }
      }
    }
  }
